vi "Shoot Cube Requested Latch.vi"(10 "Other Command Requested?":bool, 11 "Shoot Cube Pressed?":bool) -> (3 "Shoot Cube Requested?":bool)   [LabVIEW 2020]
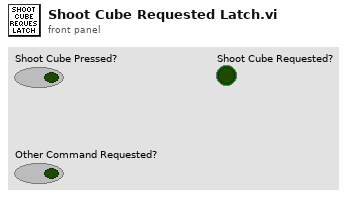
[diagram p1: front panel]
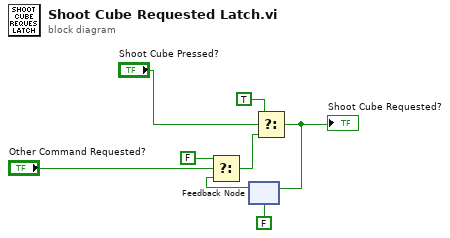
[diagram p0: block diagram]
diagram:
  n1 = feedback #1(FALSE ("t")) -> (w5:bool)
  n2 = Select(t=FALSE, s="Other Command Requested?", f=w5) -> (s? t:f=w7:bool)
  n3 = Select(t=TRUE, s="Shoot Cube Pressed?", f=w7) -> (s? t:f=w6:bool)
  "Shoot Cube Requested?" <- w6
  n4 = feedback-in #1(w6) -> ()
